vi "Worker Loop.vi"(10 "Return Queue":refnum<queue>, 11 "Application Log":refnum<class "Application Logger.lvclass">) -> ()   [LabVIEW 2019, in "Composed Log.lvlib" / "Application Logger.lvclass"]
doc: "--\nCopyright © 2017 Composed SystemsI All rights reserved.\n\nAuthor: Jon McBee <jon.mcbee@composed.io>\n\nThis library is provided \"AS IS\" ,WITHOUT WARRANTIES OR\nCONDITIONS OF ANY KIND, either express or implied.\n\nComposed Systems -- composed.io\n\nStream 0.0.1.1\nJon McBee - Composed Systems\nCopyright (c) 2017, Composed Systems"
uses:
  Application Logger.lvclass
  Types/MessageCluster.ctl
  Types/Log Packet.ctl
  Types/Log Level.ctl
  Log Sink/Log Sink.lvclass
  Application Logger.lvclass/Application Logger.ctl
  Composed Log.lvlib
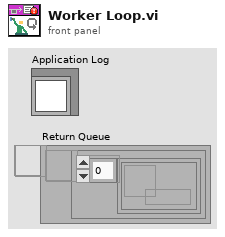
[diagram p1: front panel]
types:
  T1 = enum32{"Invalid", "Standard", "Closed", "Hidden", "Minimized", "Maximized"}
  T2 = typedef "Composed Log.lvlib/MessageCluster.ctl" = cluster{"Message":string, "Data":variant}
  T3 = typedef "Composed Log.lvlib/Log Packet.ctl" = cluster{"Data To Log":string, "Source":string, "Event Level":T4, "Event Time":timestamp}
  T4 = typedef "Composed Log.lvlib/Log Level.ctl" = enum16{"Debug", "Info", "Warning", "Error", "Critical"}
  T5 = cluster{"Log Sink":refnum<class "Log Sink.lvclass">, "queue out":refnum<queue>, "queue out":refnum<queue>}
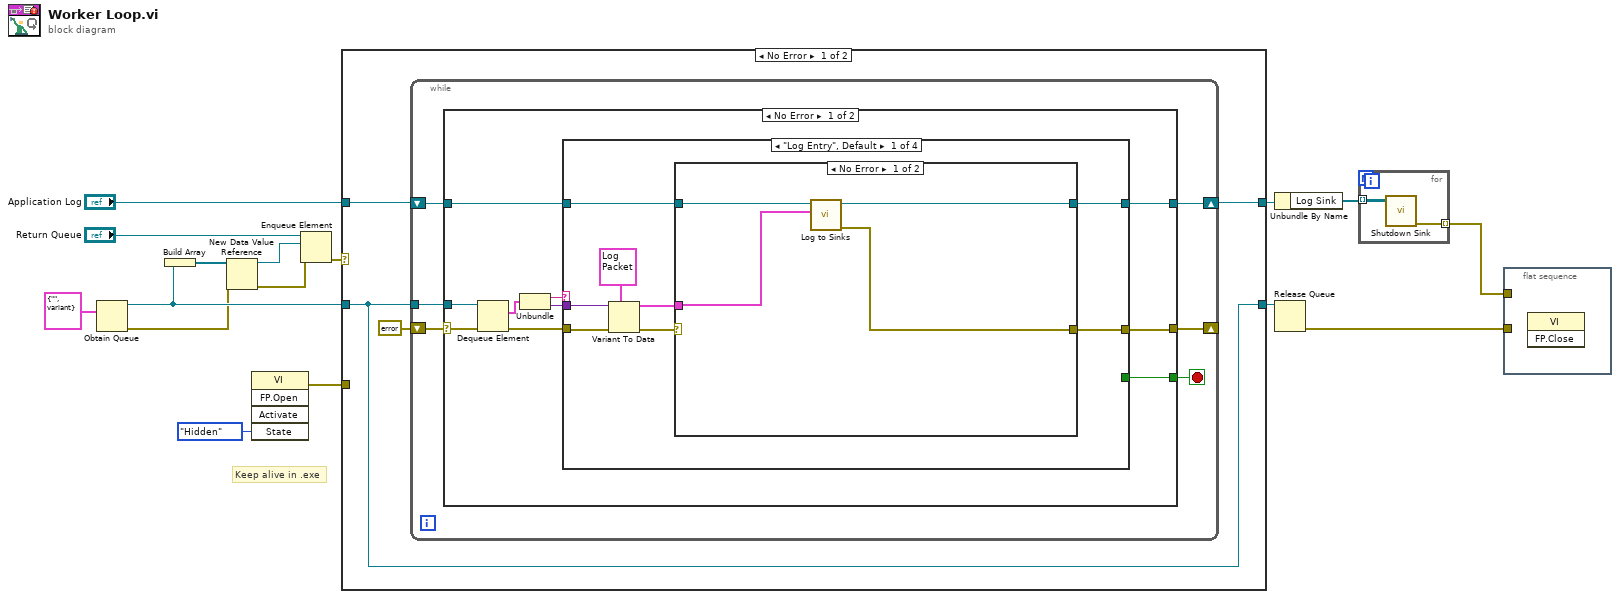
[diagram p0: block diagram]
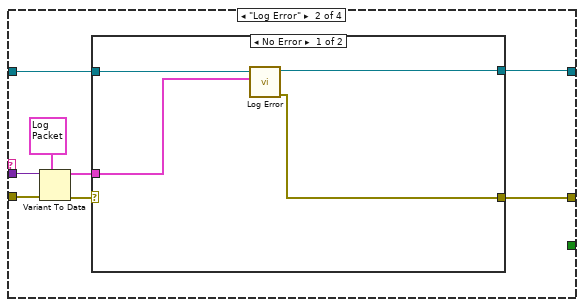
[diagram p3: hidden frame]
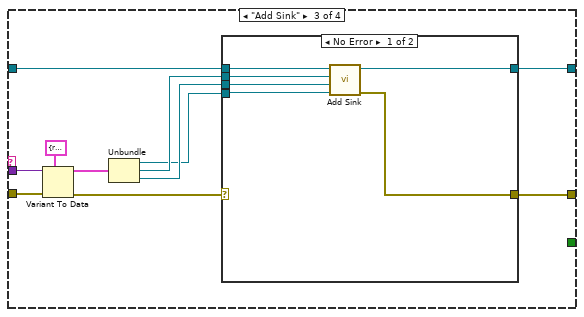
[diagram p5: hidden frame]
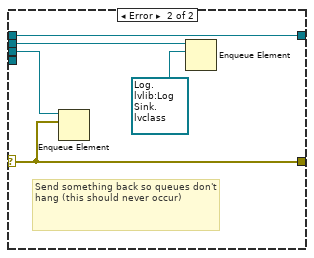
[diagram p6: hidden frame]
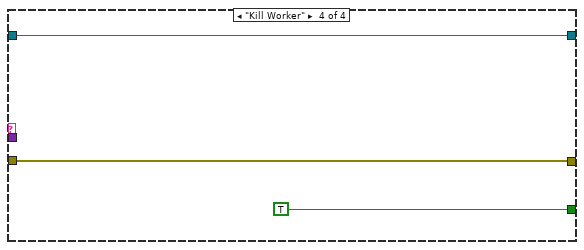
[diagram p7: hidden frame]
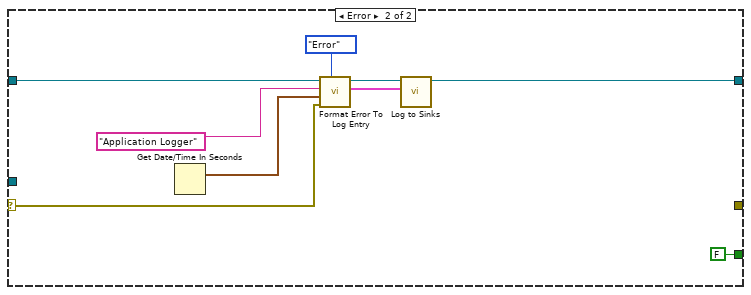
[diagram p8: hidden frame]
diagram:
  # "Keep alive in .exe"
  n1 = Obtain Queue(element data type=T2 {"Message"="", "Data"=variant}) -> (queue out=w2:refnum<queue>, error out=w1:errorcluster)  [unwired: 4 in, 1 out]
  n2 = Build Array(w2) -> (w6:refnum<queue>[])
  n3 = New Data Value Reference(data value=w6, error in=w1) -> (data value reference=w4:refnum<data-value>, error out=w3:errorcluster)
  n4 = invoke class="VI" method="FP.Open"("State"=T1."Hidden") -> (error out=w12:errorcluster)  [unwired: 4 in, 4 out]
  n5 = Enqueue Element(queue="Return Queue", element=w4, error in (no error)=w3) -> (error out=w15:errorcluster)  [unwired: 1 in, 2 out]
  n6 = case shown="No Error" w15 {
    tunnel: w2 -> [w20 w100]
    tunnel: [w20 w100] -> w14
    tunnel: "Application Log" -> [w19 w99]
    tunnel: [w18 w99] -> w8
    tunnel: w12 -> [_ _]
    frame No Error {
      n7 = while {
        tunnel: w20 -> [w26]
        shift-right: [w22] -> _
        shift-left: errorcluster {"status"=FALSE, "code"=0, "source"=""} ("error out") -> [w25]
        shift-right: [w23] -> w18
        shift-left: w19 -> [w24]
        stop <- w21 stop-if-true
        n8 = case shown="No Error" w25 {
          selector: w25 -> [w33 w92]
          tunnel: w26 -> [w34 _]
          tunnel: w24 -> [w32 w93]
          tunnel: [w31 w91] -> w23
          tunnel: [w28 _] -> w22
          tunnel: [w27 FALSE] -> w21
          frame No Error {
            n9 = Dequeue Element(queue=w34, error in (no error)=w33) -> (element=w36:T2, error out=w29:errorcluster)  [unwired: 1 in, 2 out]
            n10 = Unbundle(w36) -> ("Message"=w35:string, "Data"=w30:variant)
            n11 = case shown="\"Log Entry\", Default" w35 {
              tunnel: w32 -> [w42 w58 w74 w89]
              tunnel: [w39 w57 w73 w89] -> w31
              tunnel: w30 -> [w44 w55 w69 _]
              tunnel: w29 -> [w43 w54 w70 w88]
              tunnel: [w38 w56 w72 w88] -> w28
              tunnel: [_ _ _ TRUE] -> w27
              frame "Log Entry", Default {
                n12 = Variant To Data(error in=w43, type=T3 {"Data To Log"="", "Source"="", "Event Level"=enum."Debug", "Event Time"=timestamp(0 s since 1904-01-01)}, Variant=w44) -> (data=w40:T3, error out=w41:errorcluster)
                n13 = case shown="No Error" w41 {
                  selector: w41 -> [_ w49]
                  tunnel: w42 -> [w47 w50]
                  tunnel: w40 -> [w45 _]
                  tunnel: [w48 w50] -> w39
                  tunnel: [w46 w49] -> w38
                  frame No Error {
                    n14 = call-dynamic "Log to Sinks.vi"("Log Packet"=w45, "Asynchronous Application Log in"=w47) -> ("error out"=w46:errorcluster, "Asynchronous Application Log out"=w48:refnum<class "Application Logger.lvclass">)  [unwired: 8 in]
                  }
                  frame Error {
                  }
                }
              }
              frame "Log Error" {
                n15 = Variant To Data(error in=w54, type=T3 {"Data To Log"="", "Source"="", "Event Level"=enum."Debug", "Event Time"=timestamp(0 s since 1904-01-01)}, Variant=w55) -> (data=w52:T3, error out=w53:errorcluster)
                n16 = case shown="No Error" w53 {
                  selector: w53 -> [_ w64]
                  tunnel: w58 -> [w62 w63]
                  tunnel: [w61 w63] -> w57
                  tunnel: [w60 w64] -> w56
                  tunnel: w52 -> [w59 _]
                  frame No Error {
                    n17 = call "Log Error.vi"("Log Packet"=w59, "Application Log in"=w62) -> ("error out"=w60:errorcluster, "Application Log out"=w61:refnum<class "Application Logger.lvclass">)  [unwired: 8 in]
                  }
                  frame Error {
                  }
                }
              }
              frame "Add Sink" {
                n18 = Variant To Data(error in=w70, type=T5 {"Log Sink"=refnum, "queue out"=refnum, "queue out"=refnum} ("output cluster"), Variant=w69) -> (data=w68:T5, error out=w75:errorcluster)
                n19 = Unbundle(w68) -> ("Log Sink"=w65:refnum<class "Log Sink.lvclass">, "queue out"=w67:refnum<queue>, "queue out"=w66:refnum<queue>)
                n20 = case shown="No Error" w75 {
                  selector: w75 -> [_ w84]
                  tunnel: w67 -> [w79 w83]
                  tunnel: w66 -> [w78 w85]
                  tunnel: w65 -> [w77 _]
                  tunnel: w74 -> [w80 w86]
                  tunnel: [w81 w86] -> w73
                  tunnel: [w76 w84] -> w72
                  frame No Error {
                    n21 = call "Add Sink.vi"("Log Sink"=w77, "Error Queue"=w78, "Return Queue"=w79, "Application Logger"=w80) -> ("error out"=w76:errorcluster, "Application Logger out"=w81:refnum<class "Application Logger.lvclass">)  [unwired: 6 in]
                  }
                  frame Error {
                    # "Send something back so queues don't hang (this should never occur)"
                    n22 = Enqueue Element(queue=w85, element=w84) -> ()  [unwired: 2 in, 3 out]
                    n23 = Enqueue Element(queue=w83, element=refnum<data-value> refnum) -> ()  [unwired: 2 in, 3 out]
                  }
                }
              }
              frame "Kill Worker" {
              }
            }
          }
          frame Error {
            n24 = Get Date/Time In Seconds() -> (seconds since 1Jan1904=w94:timestamp)
            n25 = call-dynamic "Format Error To Log Entry.vi"("Event Level"=Log_Level."Error", "Error To Log"=w92, "Event Time"=w94, "Error SourceID"="Application Logger", "Application Logger In"=w93) -> ("Log Packet"=w98:T3, "Application Logger out"=w97:refnum<class "Application Logger.lvclass">)  [unwired: 5 in]
            n26 = call-dynamic "Log to Sinks.vi"("Log Packet"=w98, "Asynchronous Application Log in"=w97) -> ("Asynchronous Application Log out"=w91:refnum<class "Application Logger.lvclass">)  [unwired: 8 in, 1 out]
          }
        }
      }
    }
    frame Error {
      # "If returning the queue reference returns an error, just stop - we would have no way to stop the daemon otherwise! (This should never occur)"
    }
  }
  n27 = Unbundle By Name(w8) -> ("Log Sink"=w9:refnum<data-value>[])
  n28 = Release Queue(queue=w14) -> (error out=w11:errorcluster)  [unwired: 2 in, 2 out]
  n29 = for {
    tunnel: w9 -> [w102] mode=indexing
    tunnel: [w101] -> w7 mode=indexing
    n30 = call "Shutdown Sink.vi"("Log Sink"=w102) -> ("error out"=w101:errorcluster)  [unwired: 10 in]
  }
  n31 = flat-sequence {
    tunnel: w11 -> [_]
    tunnel: w7 -> [_]
    frame #0 {
      n32 = invoke class="VI" method="FP.Close"() -> ()  [unwired: 3 in, 3 out]
    }
  }
